vi "Close All Page.vi"(8 "error in (no error)":errorcluster, 11 "QTab Class in":refnum<class "QTab Class.lvclass">) -> (0 "error out":errorcluster, 2 "VI Refnum []":refnum<vi>[](array[refnum]), 3 "QTab Class out":refnum<class "QTab Class.lvclass">)   [LabVIEW 2020, in "QTab.lvlib" / "QTab Class.lvclass"]
uses:
  QTab Class.lvclass
  Command.ctl
  QTab Class.lvclass/QTab Class.ctl
  Pag Attribute.ctl
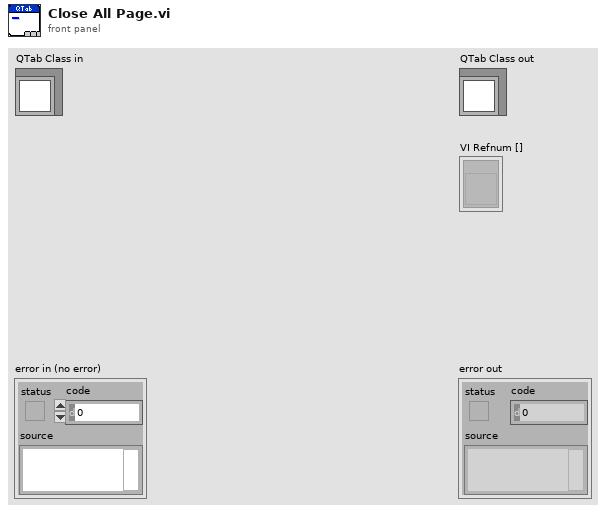
[diagram p1: front panel]
types:
  T1 = typedef "QTab.lvlib/QTab Class.lvclass/Command.ctl" = enum16{"Startup", "Add Page", "Close All Page", "Set Page Attribute", "Pop-out", "Merage", "Insert", "Stop"}
  T2 = typedef "QTab.lvlib/QTab Class.lvclass/Pag Attribute.ctl" = cluster{"VI Refnum":refnum<vi>, "Page Name":string, "Closeable":bool, "Draggable":bool, "Pop-Out":bool}
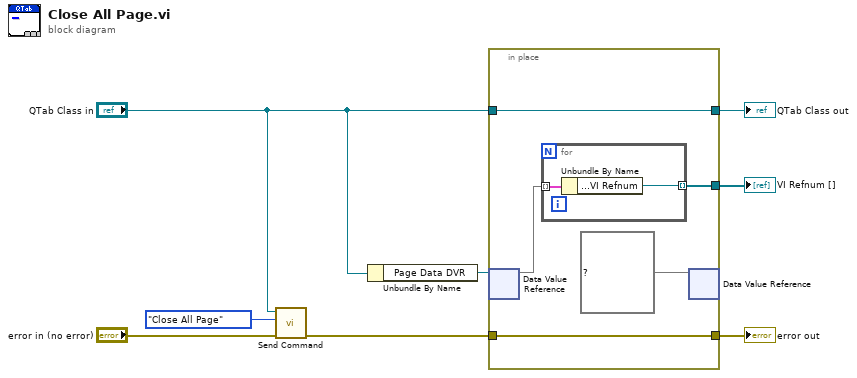
[diagram p0: block diagram]
diagram:
  n1 = call "Send Command.vi"("error in (no error)"="error in (no error)", "Command"=Command."Close All Page", "QTab Class in"="QTab Class in") -> ("error out"=w3:errorcluster)  [unwired: 7 in, 1 out]
  n2 = Unbundle By Name("QTab Class in") -> ("Page Data DVR"=w6:refnum<data-value>)
  n3 = in-place {
    in-place-border: "QTab Class in" -> [w13]
    in-place-border: [w13] -> w4
    in-place-border: w3 -> [w12]
    in-place-border: [w12] -> w2
    in-place-border: [w10] -> w1
    n4 = in-place-dvr #1(w6) -> (w11:map{string, T2})  [unwired: 1 out]
    n5 = for {
      tunnel: w11 -> [w15] mode=indexing
      tunnel: [w14] -> w10 mode=indexing
      n6 = Unbundle By Name(w15) -> ("Pag Attribute.VI Refnum"=w14:refnum<vi>)
    }
    n7 = in-place-dvr #1(map{string, T2} {} ("data value")) -> ()  [unwired: 2 out]
  }
  "error out" <- w2
  "QTab Class out" <- w4
  "VI Refnum []" <- w1
